vi "多设备同步_外部触发源.vi"() -> ()   [LabVIEW 2013]
uses:
  <userlib>/ArtDAQ/_SubVI/ArtDAQ_CreateAIVoltageChan.vi
  <userlib>/ArtDAQ/_SubVI/ArtDAQ_CfgSampClkTiming.vi
  <userlib>/ArtDAQ/_SubVI/ArtDAQ_CfgDigEdgeStartTrig.vi
  <userlib>/ArtDAQ/_SubVI/ArtDAQ_Read Analog DBL NChan NSamp.vi
panel:
  out "?":dbl[][](graph)
  out "?":dbl[][](graph)
  in  "Stop":bool
  in  "物理通道2":string(combo)="Dev2/ai0"
  in  "物理通道1":string(combo)="Dev1/ai0"
  out "ErrorOutput":errorcluster
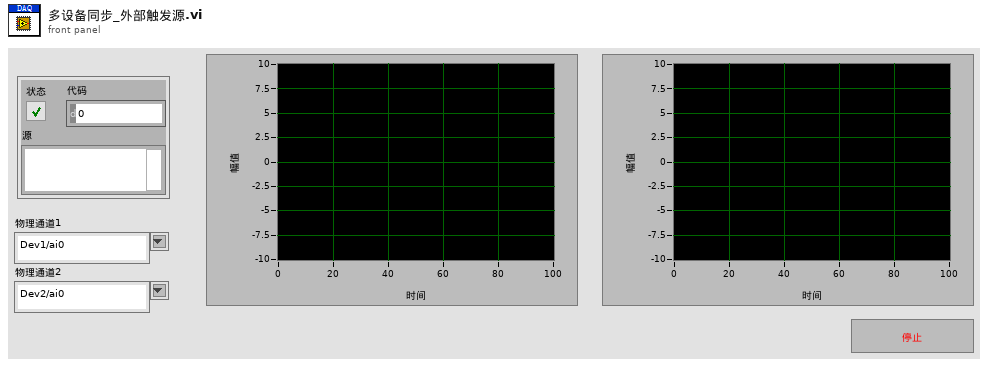
[diagram p1: front panel]
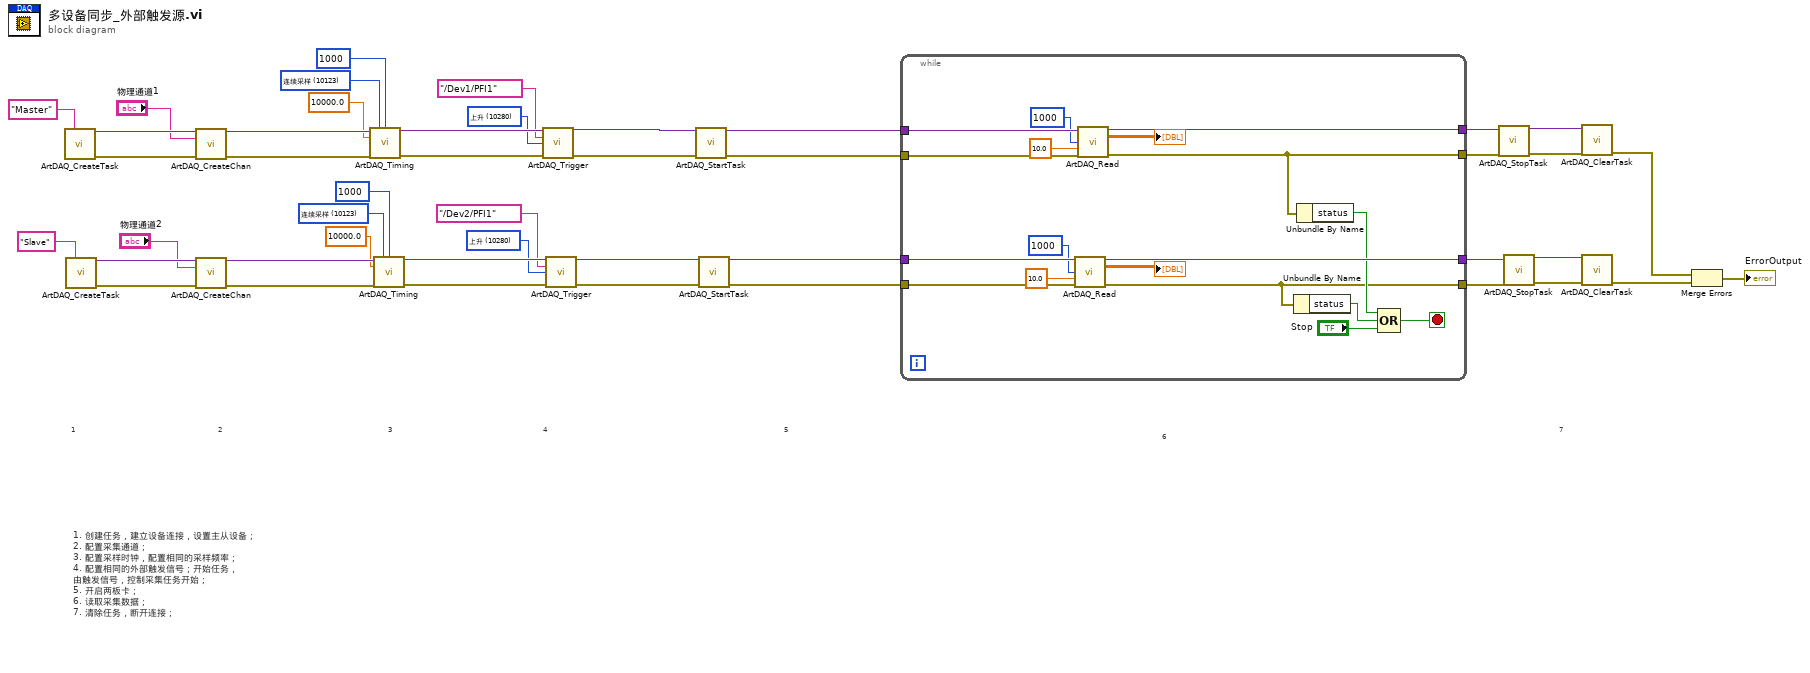
[diagram p0: block diagram]
diagram:
  w1 = 10280 items=["上升"=10280, "下降"=10171] ("有效边沿")
  w4 = 10280 items=["上升"=10280, "下降"=10171] ("有效边沿")
  w13 = 10123 items=["有限点采样"=10178, "连续采样"=10123] ("采样模式")
  w14 = 10123 items=["有限点采样"=10178, "连续采样"=10123, "硬件定时单点"=12522, "软件定时单点"=12523] ("SampleMode")
  # "1. 创建任务，建立设备连接，设置主从设备；\n2. 配置采集通道；\n3. 配置采样时钟，配置相同的采样频率；\n4. 配置相同的外部触发信号；开始任务，\n由触发信号，控制采集任务开始；\n5. 开启两板卡；\n6. 读取采集数据；\n7. 清除任务，断开连接；"
  # "7"
  # "6"
  # "5"
  # "4"
  # "3"
  # "2"
  # "1"
  n1 = call <userlib>:"ArtDAQ_CreateTask.vi"("任务名称"="Master" ("TaskName")) -> ("任务句柄"=w45:variant, "错误输出"=w44:errorcluster)  [unwired: 13 in]
  n2 = call <userlib>:"ArtDAQ_CreateTask.vi"("任务名称"="Slave" ("TaskName")) -> ("任务句柄"=w43:variant, "错误输出"=w42:errorcluster)  [unwired: 13 in]
  n3 = call-poly <userlib>:"ArtDAQ_CreateChan.vi"("任务句柄"=w45, "物理通道"="物理通道1", "错误输入"=w44) -> ("任务句柄"=w41:variant, "错误输出"=w40:errorcluster)  [unwired: 11 in]
  n4 = call-poly <userlib>:"ArtDAQ_CreateChan.vi"("任务句柄"=w43, "物理通道"="物理通道2", "错误输入"=w42) -> ("任务句柄"=w39:variant, "错误输出"=w38:errorcluster)  [unwired: 11 in]
  n5 = call-poly <userlib>:"ArtDAQ_Timing.vi"("任务句柄"=w41, "采样模式"=w14, "每通道采样数"=1000 ("SamplePerChan"), "采样率"=10000.0 ("Rate"), "错误输入"=w40) -> ("任务句柄"=w10:variant, "错误输出"=w9:errorcluster)  [unwired: 9 in]
  n6 = call-poly <userlib>:"ArtDAQ_Timing.vi"("任务句柄"=w39, "采样模式"=w13, "每通道采样数"=1000 ("SamplePerChan"), "采样率"=10000.0 ("Rate"), "错误输入"=w38) -> ("任务句柄"=w8:variant, "错误输出"=w6:errorcluster)  [unwired: 9 in]
  n7 = call-poly <userlib>:"ArtDAQ_Trigger.vi"("任务句柄"=w10, "触发源"="/Dev1/PFI1" ("TriggerSource"), "边沿"=w4, "错误输入"=w9) -> ("任务句柄"=w37:variant, "错误输出"=w36:errorcluster)  [unwired: 10 in]
  n8 = call-poly <userlib>:"ArtDAQ_Trigger.vi"("任务句柄"=w8, "触发源"="/Dev2/PFI1" ("TriggerSource"), "边沿"=w1, "错误输入"=w6) -> ("任务句柄"=w7:variant, "错误输出"=w5:errorcluster)  [unwired: 10 in]
  n9 = call <userlib>:"ArtDAQ_StartTask.vi"("任务句柄"=w37, "错误输入"=w36) -> ("任务句柄"=w35:variant, "错误输出"=w34:errorcluster)  [unwired: 12 in]
  n10 = call <userlib>:"ArtDAQ_StartTask.vi"("任务句柄"=w7, "错误输入"=w5) -> ("任务句柄"=w33:variant, "错误输出"=w32:errorcluster)  [unwired: 12 in]
  n11 = while {
    tunnel: w35 -> [w63]
    tunnel: w34 -> [w62]
    tunnel: w33 -> [w61]
    tunnel: w32 -> [w60]
    tunnel: [w59] -> w31
    tunnel: [w54] -> w30
    tunnel: [w58] -> w29
    tunnel: [w52] -> w28
    stop <- w55 stop-if-true
    n12 = call-poly <userlib>:"ArtDAQ_Read.vi"("任务句柄"=w61, "每通道采样数"=1000 ("NumSampsPerChan"), "超时s"=10.0 ("Timeout"), "错误输入"=w60) -> ("任务句柄"=w58:variant, "数据"=→"?":dbl[][], "错误输出"=w52:errorcluster)  [unwired: 7 in, 2 out]
    n13 = call-poly <userlib>:"ArtDAQ_Read.vi"("任务句柄"=w63, "每通道采样数"=1000 ("NumSampsPerChan"), "超时s"=10.0 ("Timeout"), "错误输入"=w62) -> ("任务句柄"=w59:variant, "数据"=→"?":dbl[][], "错误输出"=w54:errorcluster)  [unwired: 7 in, 2 out]
    n14 = Unbundle By Name(w52) -> ("status"=w51:bool)
    n15 = Unbundle By Name(w54) -> ("status"=w53:bool)
    n16 = Compound Arithmetic op=OR(w53, w51, "Stop") -> (w55:bool)
  }
  n17 = call <userlib>:"ArtDAQ_StopTask.vi"("任务句柄"=w31, "错误输入"=w30) -> ("任务句柄"=w27:variant, "错误输出"=w26:errorcluster)  [unwired: 12 in]
  n18 = call <userlib>:"ArtDAQ_StopTask.vi"("任务句柄"=w29, "错误输入"=w28) -> ("任务句柄"=w25:variant, "错误输出"=w24:errorcluster)  [unwired: 12 in]
  n19 = call <userlib>:"ArtDAQ_ClearTask.vi"("任务句柄"=w27, "错误输入"=w26) -> ("错误输出"=w23:errorcluster)  [unwired: 13 in]
  n20 = call <userlib>:"ArtDAQ_ClearTask.vi"("任务句柄"=w25, "错误输入"=w24) -> ("错误输出"=w22:errorcluster)  [unwired: 13 in]
  n21 = Merge Errors(w23, w22) -> (→"ErrorOutput":errorcluster)
